vi "Door Closed Interlock Value Change.vi"(8 "error in (no error)":errorcluster, 10 "Door Closed Interlock":bool, 11 "Doors Closing in":refnum<class "Doors Closing.lvclass">) -> (0 "error out":errorcluster, 3 "Doors Closing out":refnum<class "Doors Closing.lvclass">)   [LabVIEW 2020, in "Door Controller.lvlib" / "Doors Closing.lvclass"]
uses:
  Doors Closing.lvclass
  C:/Users/Thomas.McQuillan/Desktop/Elevator Door Control/Door Controller/Door Controller/Door Controller.lvclass
  Application/Application/Interlock Names.ctl
  Door Controller/Door Controller.lvclass/Door Controller.ctl
  <vilib>/ActorFramework/Message Enqueuer/Message Enqueuer.lvclass/Message Enqueuer.ctl
  <vilib>/ActorFramework/Message Enqueuer/Enqueue.vi
  Door Hardware/Door Hardware Messages/Stop Door Actuators Msg/Stop Door Actuators Msg.lvclass
  C:/Program Files/National Instruments/LabVIEW 2020/vi.lib/ActorFramework/Message/Message.lvclass
  <vilib>/ActorFramework/Message Priority Queue/Priority Enqueue.vi
  Door Controller/Door Controller.lvclass
  Application/Application.lvlib
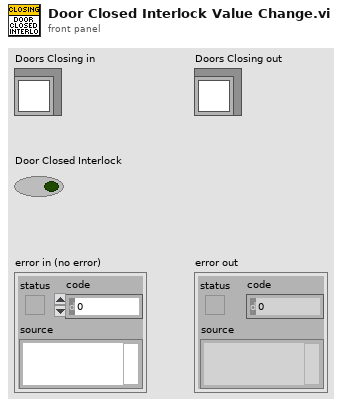
[diagram p1: front panel]
types:
  T1 = typedef "Application.lvlib/Interlock Names.ctl" = enum16{"Door Closed Interlock", "Door Open Interlock"}
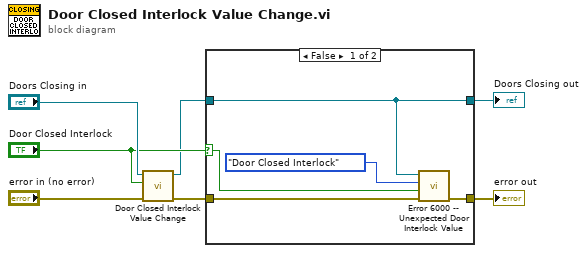
[diagram p0: block diagram]
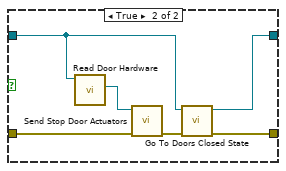
[diagram p2: hidden frame]
diagram:
  n1 = call-parent "Door Closed Interlock Value Change.vi"("error in (no error)"="error in (no error)", "Door Closed Interlock"="Door Closed Interlock", "Door Controller in"="Doors Closing in") -> ("error out"=w1:errorcluster, "Door Controller out"=w4:refnum<class "Doors Closing.lvclass">)  [unwired: 7 in]
  n2 = case shown="False" "Door Closed Interlock" {
    selector: "Door Closed Interlock" -> [w8 _]
    tunnel: w4 -> [w11 w16]
    tunnel: [w11 w15] -> w3
    tunnel: [w9 w14] -> w2
    tunnel: w1 -> [w10 w17]
    frame False {
      n3 = call "Error 6000 -- Unexpected Door Interlock Value.vi"("error in (no error)"=w10, "Interlock Value"=w8, "Interlock Name"=Interlock_Names."Door Closed Interlock", "Door Controller"=w11) -> ("error out"=w9:errorcluster)  [unwired: 7 in]
    }
    frame True {
      n4 = call "Read Door Hardware.vi"("Door Controller in"=w16) -> ("Door Hardware"=w18:refnum<class "Message Enqueuer.lvclass">)  [unwired: 10 in]
      n5 = call "Send Stop Door Actuators.vi"("error in (no error)"=w17, "Message Enqueuer"=w18) -> ("error out"=w13:errorcluster)  [unwired: 8 in, 1 out]
      n6 = call "Go To Doors Closed State.vi"("error in (no error)"=w13, "Door Controller in"=w16) -> ("error out"=w14:errorcluster, "Door Controller out"=w15:refnum<class "Doors Closing.lvclass">)  [unwired: 8 in]
    }
  }
  "error out" <- w2
  "Doors Closing out" <- w3
